vi "Main - TTU Swarm Field.vi"() -> (0 "Error Cluster":errorcluster, 3 "Field Processing Result":T2(plugin-control))   [LabVIEW 2018]
uses:
  <vilib>/userdefined/High Color/IMAQdx.ctl
  <vilib>/vision/driver/IMAQdx.llb/IMAQdx Camera Control Mode.ctl
  <vilib>/myRIO/Instrument Drivers/Onboard IO/DIO/typedefs/DIO Reference.ctl
  <vilib>/myRIO/Common/Instrument Driver Framework/Utilities/typedefs/myRIO Generic Hardware Reference.ctl
  <vilib>/myRIO/Common/Instrument Driver Framework/Utilities/typedefs/Hardware Version Enum.ctl
  <vilib>/myRIO/Common/Instrument Driver Framework/Utilities/typedefs/myRIO v1.0 Reference.ctl
  <vilib>/myRIO/Common/Instrument Driver Framework/Utilities/typedefs/Generic FPGA Reference.ctl
  <vilib>/myRIO/Common/Instrument Driver Framework/myRIO v1.0/DIO/typedefs/DIO Channels List.ctl
  <vilib>/myRIO/Common/Instrument Driver Framework/myRIO v1.0/DIO/typedefs/DIO Channels Enum.ctl
  <vilib>/userdefined/High Color/nirio_resource_hc.ctl
  <vilib>/myRIO/Common/Instrument Driver Framework/Utilities/vis/Is FPGA Ref Available.vi
  <vilib>/myRIO/Common/Instrument Driver Framework/myRIO v1.0/DIO/vis/myRIO v1.1 Open DIO.vi
  <vilib>/myRIO/Instrument Drivers/Onboard IO/DIO/vis/Write.vi
  <vilib>/myRIO/Common/Instrument Driver Framework/Utilities/vis/Validate Channels.vi
  <vilib>/myRIO/Common/Instrument Driver Framework/myRIO v1.0/DIO/vis/myRIO v1.0 Reserve DIO.vi
  <vilib>/myRIO/Common/Instrument Driver Framework/myRIO v1.0/Resource Manager/vis/myRIO v1.0 Reserve Channel List.vi
  <vilib>/myRIO/Common/Instrument Driver Framework/myRIO v1.0/DIO/vis/myRIO v1.0 Build MUX Configuration DIO.vi
  <vilib>/myRIO/Common/Instrument Driver Framework/myRIO v1.0/Resource Manager/vis/myRIO v1.0 Reserve Channel.vi
  <vilib>/myRIO/Common/Instrument Driver Framework/myRIO v1.0/Resource Manager/vis/myRIO v1.0 Unreserve Channel.vi
  <vilib>/myRIO/Common/Instrument Driver Framework/myRIO v1.0/Resource Manager/vis/myRIO v1.0 Create Configuration List.vi
  <vilib>/myRIO/Common/Instrument Driver Framework/myRIO v1.0/Resource Manager/vis/myRIO v1.0 Build Mutex Name.vi
  <vilib>/Utility/VariantDataType/GetNumericInfo.vi
  <vilib>/Utility/error.llb/Error Cluster From Error Code.vi
  <vilib>/myRIO/Common/Instrument Driver Framework/myRIO v1.0/myRIO v1.1 Open.vi
  <vilib>/myRIO/Common/Instrument Driver Framework/Utilities/vis/IO Manager.vi
  <vilib>/myRIO/Common/Instrument Driver Framework/Utilities/vis/Configuration Manager.vi
  <vilib>/myRIO/Common/Instrument Driver Framework/myRIO v1.0/Resource Manager/vis/myRIO v1.0 Configure IO.vi
  <vilib>/myRIO/Common/Instrument Driver Framework/myRIO v1.0/myRIO v1.0 Close.vi
  <vilib>/myRIO/Common/Instrument Driver Framework/myRIO v1.0/DIO/vis/myRIO v1.0 Write DIO.vi
  <vilib>/myRIO/Express VI/Onboard Devices/LED/LED Express VI.xnode
  <vilib>/myRIO/Instrument Drivers/Onboard IO/DIO/vis/myRIO DIO Open.xnode
  <vilib>/vision/driver/NI_Vision_Acquisition_Software.lvlib
  <vilib>/myRIO/Instrument Drivers/Onboard IO/DIO/DIO.lvlib
panel:
  out "Frequency (Hz)":dbl
  in  "Stop Button":bool
  in  "Exposure":i64(slide)=791 min=41 max=10000 step=50 scale=41.0..2000.0 scale format="%#_6p"
  in  "Brightness":i64(slide) min=-64 max=64 step=1 scale=-64.0..64.0
  in  "Contrast":i64(slide)=53 min=0 max=100 step=1 scale=0.0..100.0
  in  "Gain":i64(slide)=49 min=0 max=128 step=1 scale=0.0..128.0
  in  "Camera":T1="cam1"
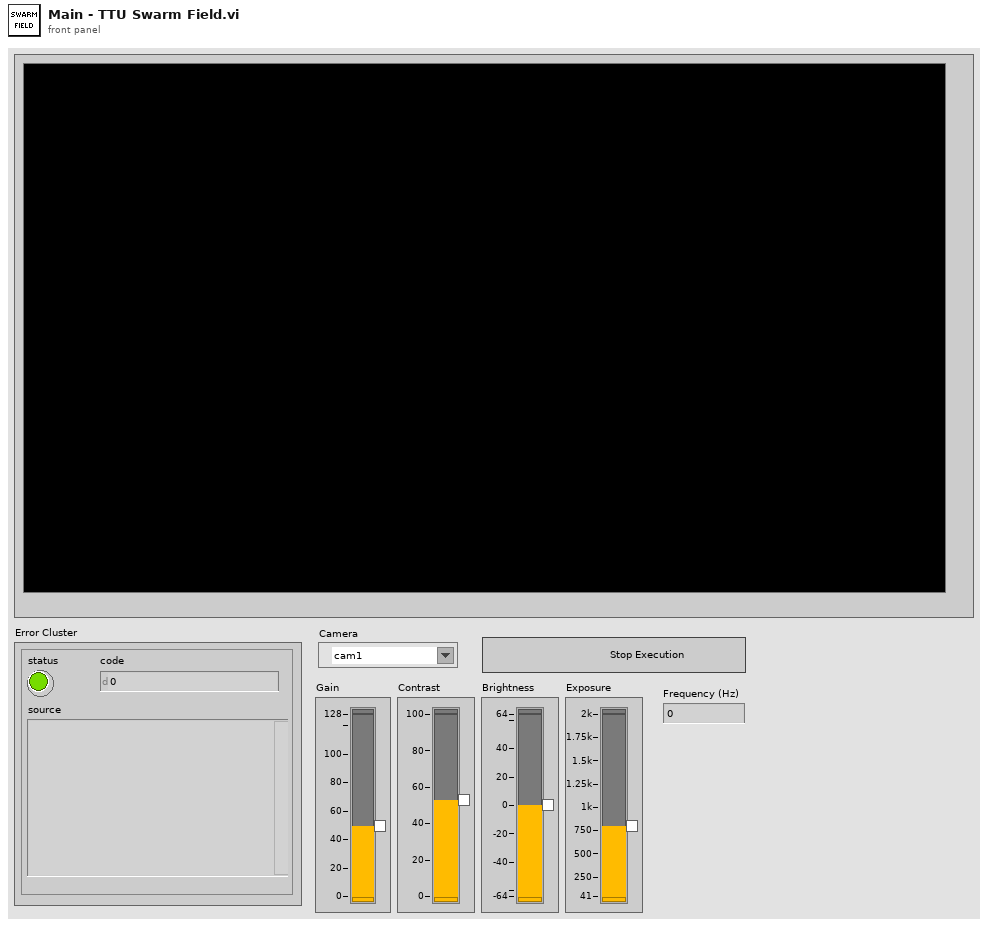
[diagram p1: front panel]
types:
  T1 = typedef "IMAQdx.ctl" = refnum<k21>
  T2 = typedef "IMAQ Image.ctl" = refnum<image>
  T3 = typedef "NI_Vision_Acquisition_Software.lvlib/IMAQdx Camera Control Mode.ctl" = enum32{"Controller", "Listener"}
  T4 = typedef "DIO.lvlib/DIO Reference.ctl" = cluster{"myRIO Reference":T5, "DIO Channels List":T9}
  T5 = typedef "myRIO Generic Hardware Reference.ctl" = cluster{"myRIO Model":T6, "myRIO Hardware Reference":T7}
  T6 = typedef "Hardware Version Enum.ctl" = enum16{"Unknown", "myRIO-1900", "myRIO-1950", "roboRIO", "NI ELVIS RIO CM", "ELVIS III"}
  T7 = typedef "myRIO v1.0 Reference.ctl" = cluster{"Generic FPGA Reference":T8, "Allow multiple opens":bool}
  T8 = typedef "Generic FPGA Reference.ctl" = refnum<k20>
  T9 = typedef "DIO Channels List.ctl" = T10[]
  T10 = typedef "DIO Channels Enum.ctl" = enum16{"Not Connected", "C/DIO0", "C/DIO1", "C/DIO2", "C/DIO3", "C/DIO4", "C/DIO5", "C/DIO6", "C/DIO7", "A/DIO0", "A/DIO1", "A/DIO2", "A/DIO3", "A/DIO4", "A/DIO5", "A/DIO6", "A/DIO7", "A/DIO8", "A/DIO9", "A/DIO10", "A/DIO11", "A/DIO12", "A/DIO13", "A/DIO14", "A/DIO15", "A/DIO16", "A/DIO17", "A/DIO18", "A/DIO19", "B/DIO0", "B/DIO1", "B/DIO2", "B/DIO3", "B/DIO4", "B/DIO5", "B/DIO6", "B/DIO7", "B/DIO8", "B/DIO9", "B/DIO10", "B/DIO11", "B/DIO12", "B/DIO13", "B/DIO14", "B/DIO15", "B/DIO16", "B/DIO17", "B/DIO18", "B/DIO19", "LED0", "LED1", "LED2", "LED3", "Button0", "DIO/DIO0", "DIO/DIO1", "DIO/DIO2", "DIO/DIO3", "DIO/DIO4", "DIO/DIO5", "DIO/DIO6", "DIO/DIO7", "DIO/DIO8", "DIO/DIO9", "SPI/CS0", "SPI/CS1", "SPI/CS2", "SPI/CS3", "LED RADIO (Green)", "LED RADIO (Red)", "LED COMM (Green)", "LED COMM (Red)", "LED MODE (Green)", "LED MODE (Red)"}
  T11 = typedef "nirio_resource_hc.ctl" = tag
  T12 = typedef "Image Object.ctl" = cluster{"Objects":cluster{"Object Center":cluster{"X":sgl, "Y":sgl}, "Bounding Box":cluster{"X Left":i32, "Y Top":i32, "X Right":i32, "Y Bottom":i32}, "Area":sgl, "Orientation":sgl, "Aspect Ratio":sgl, "Nb Holes":i32}[], "Image":T2}
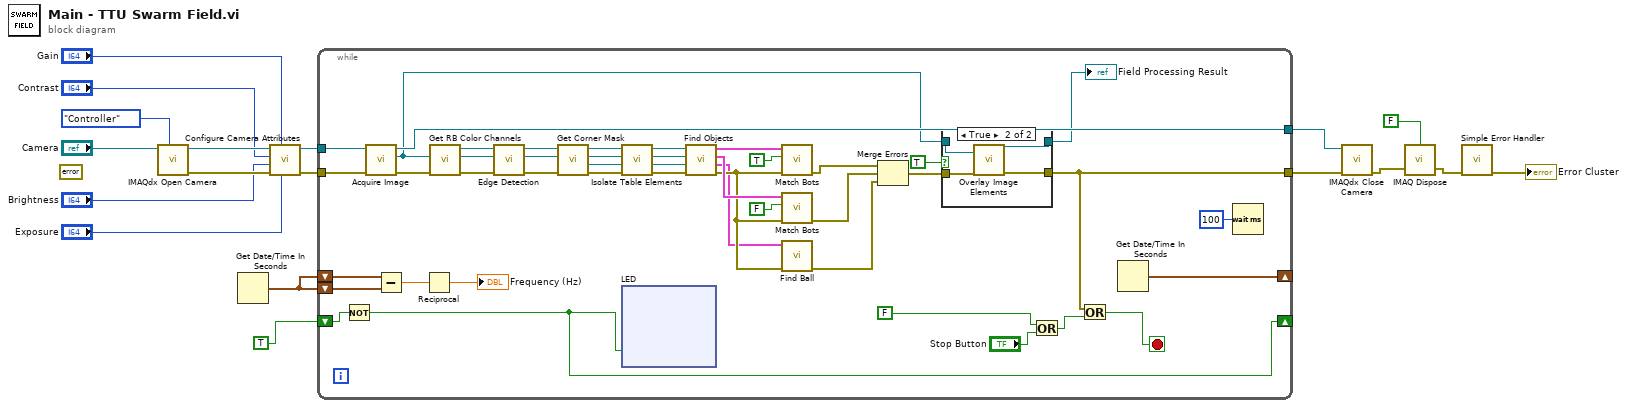
[diagram p0: block diagram]
diagram:
  (unwired) errorcluster {"status"=FALSE, "code"=0, "source"=""} ("error in")
  n1 = call <vilib>:"IMAQdx Open Camera.vi"("Camera Control Mode"=IMAQdx_Camera_Control_Mode."Controller", "Session In"="Camera") -> ("error out"=w17:errorcluster, "Session Out"=w16:T1)  [unwired: 8 in]
  n2 = Get Date/Time In Seconds() -> (seconds since 1Jan1904=w5:timestamp)
  n3 = call "Configure Camera Attributes.vi"("Exposure"="Exposure", "Gain"="Gain", "Error In"=w17, "Brightness"="Brightness", "Contrast"="Contrast", "Camera In"=w16) -> ("Error Out"=w11:errorcluster, "Camera Out"=w10:T1)  [unwired: 4 in]
  n4 = while {
    tunnel: w11 -> [w62]
    tunnel: w10 -> [w61]
    tunnel: [w42] -> w9
    tunnel: [w50] -> w8
    shift-right: [w56] -> _
    shift-left: w5 -> [w55]
    shift-left: w5 -> [w54]
    shift-right: [w20] -> _
    shift-left: TRUE -> [w21]
    stop <- w57 stop-if-true
    n5 = Not(x=w21) -> (.not. x?=w20:bool)
    n6 = call "Acquire Image.vi"("Error In"=w62, "Camera In"=w61) -> ("Error Out"=w51:errorcluster, "Image"=w43:T2, "Camera Out"=w50:T1)  [unwired: 7 in]
    n7 = Subtract(x=w54, y=w55) -> (x-y=w53:dbl)
    n8 = Reciprocal(x=w53) -> (1/x=→"Frequency (Hz)":dbl)
    n9 = call "Get RB Color Channels.vi"("Error In"=w51, "Image In"=w43) -> ("Error Out"=w49:errorcluster, "Blue Channel"=w48:T2, "Red Channel"=w47:T2)  [unwired: 7 in]
    n10 = call "Edge Detection.vi"("Error In"=w49, "Blue Channel"=w48, "Red Channel"=w47) -> ("Error Out"=w46:errorcluster, "Blue Edges"=w45:T2, "Red Edges"=w44:T2)  [unwired: 6 in]
    n11 = call "Get Corner Mask.vi"("Error In"=w46, "Blue Channel In"=w45, "Red Channel In"=w44) -> ("Error Out"=w41:errorcluster, "Corner Mask"=w40:T2, "Blue Channel Out"=w39:T2, "Red Channel Out"=w38:T2)  [unwired: 5 in]
    n12 = call "Isolate Table Elements.vi"("Error In"=w41, "Corner Mask"=w40, "Blue Channel In"=w39, "Red Channel In"=w38) -> ("Error Out"=w37:errorcluster, "Game Ball"=w36:T2, "Blue Team"=w35:T2, "Red Team"=w34:T2)  [unwired: 4 in]
    n13 = xnode "LED"("LED0"=w20) -> ()  [unwired: 1 in, 1 out]
    n14 = call "Find Objects.vi"("Error In"=w37, "Game Ball"=w36, "Blue Team"=w35, "Red Team"=w34) -> ("Error Out"=w25:errorcluster, "Ball Object"=w24:T12, "Blue Objects"=w29:T12, "Red Objects"=w32:T12)  [unwired: 4 in]
    n15 = call "Match Bots.vi"("Error In"=w25, "isRed"=TRUE, "Image Objects"=w32) -> ("Error Out"=w28:errorcluster)  [unwired: 8 in]
    n16 = call "Match Bots.vi"("Error In"=w25, "isRed"=FALSE, "Image Objects"=w29) -> ("Error Out"=w27:errorcluster)  [unwired: 8 in]
    n17 = call "Find Ball.vi"("Error In"=w25, "Ball Object"=w24) -> ("Error Out"=w23:errorcluster)  [unwired: 9 in]
    n18 = Merge Errors(w28, w27, w23) -> (w26:errorcluster)
    n19 = case shown="True" TRUE {
      tunnel: w43 -> [w99 w103]
      tunnel: [w98 w102] -> w42
      tunnel: [w99 w101] -> w33
      tunnel: w26 -> [w98 w100]
      frame False {
      }
      frame True {
        n20 = call "Overlay Image Elements.vi"("Image In"=w103, "Error In"=w100) -> ("Error Out"=w102:errorcluster, "Overlayed Image"=w101:T2)  [unwired: 8 in]
      }
    }
    "Field Processing Result" <- w33
    n21 = Or(x=FALSE, y="Stop Button") -> (x .or. y?=w58:bool)
    n22 = Or(x=w42, y=w58) -> (x .or. y?=w57:bool)
    n23 = Get Date/Time In Seconds() -> (seconds since 1Jan1904=w56:timestamp)
    n24 = Wait (ms)(milliseconds to wait=u32 100) -> ()  [unwired: 1 out]
  }
  n25 = call <vilib>:"IMAQdx Close Camera.vi"("error in"=w9, "Session In"=w8) -> ("error out"=w3:errorcluster)  [unwired: 9 in]
  n26 = call "IMAQ Dispose"("All Images? (No)"=FALSE, "error in (no error)"=w3) -> ("error out"=w2:errorcluster)  [unwired: 4 in]
  n27 = call <vilib>:"Simple Error Handler.vi"("error in (no error)"=w2) -> ("error out"=→"Error Cluster":errorcluster)  [unwired: 4 in, 4 out]
